vi "Stop_Video.vi"(0 "VLC Variables In":T1, 11 "error in (no error)":errorcluster) -> (15 "error out":errorcluster)   [LabVIEW 2012]
doc: "Stop streaming video"
uses:
  Controls-Webcam/VLC Var.ctl
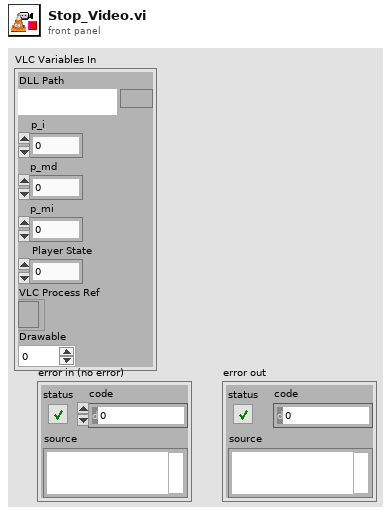
[diagram p1: front panel]
types:
  T1 = typedef "VLC Var.ctl" = cluster{"DLL Path":path, "p_i":i32, "p_md":i32, "p_mi":i32, "Player State":i32, "VLC Process Ref":refnum<k24>, "Drawable":i32}
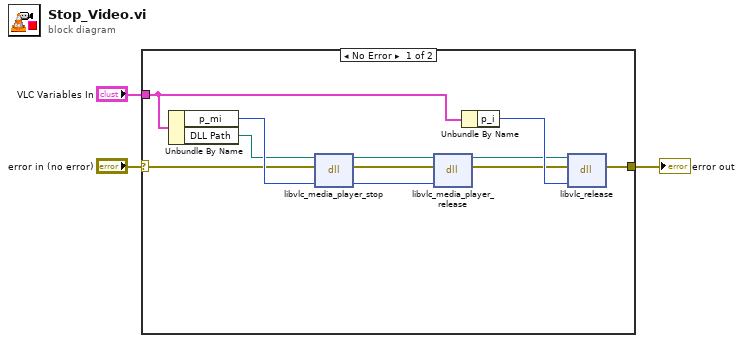
[diagram p0: block diagram]
diagram:
  n1 = case shown="No Error" "error in (no error)" {
    selector: "error in (no error)" -> [w5 w15]
    tunnel: "VLC Variables In" -> [w14 _]
    tunnel: [w13 w15] -> w2
    frame No Error {
      n2 = Unbundle By Name(w14) -> ("p_mi"=w8:i32, "DLL Path"=w4:path)
      n3 = dll-call lib="C:/Program Files (x86)/VideoLAN/VLC/libvlc.dll" fn="libvlc_media_player_stop"(path in=w4, error in=w5, "p_mi"=w8) -> (path out=w6:path, error out=w7:errorcluster, "p_mi"=w9:i32)  [unwired: 2 in]
      n4 = dll-call lib="C:/Program Files (x86)/VideoLAN/VLC/libvlc.dll" fn="libvlc_media_player_release"(path in=w6, error in=w7, "p_mi"=w9) -> (path out=w11:path, error out=w10:errorcluster)  [unwired: 3 in]
      n5 = Unbundle By Name(w14) -> ("p_i"=w12:i32)
      n6 = dll-call lib="C:/Program Files (x86)/VideoLAN/VLC/libvlc.dll" fn="libvlc_release"(path in=w11, error in=w10, "p_instnace"=w12) -> (error out=w13:errorcluster)  [unwired: 3 in, 1 out]
    }
    frame Error {
    }
  }
  "error out" <- w2
